vi "Write Error Log.vi"(5 "system directory type":T1=1 items=["User Home"=0, "User Desktop"=1, "User Documents"=2, "User Application Data"=3, "User Preferences"=4, "User Temporary"=5, "Public Documents"=6, "Public Application Data"=7, "Public Preferences"=8, "Public Cache"=13, "System Core Libraries"=9, "System Installed Libraries"=10, "Application Files"=11, "Boot Volume Root"=12], 6 "Thread":string, 7 "error IO":errorcluster, 9 "Additional info":string) -> (0 "error out":errorcluster)   [LabVIEW 2017]
uses:
  <vilib>/Utility/sysdir.llb/System Directory Type.ctl
  <vilib>/Utility/error.llb/DialogType.ctl
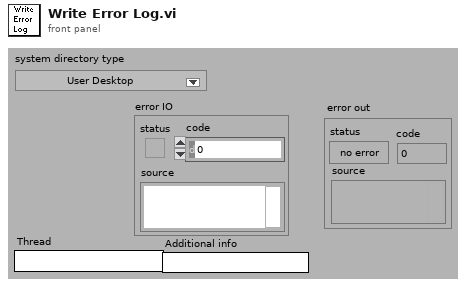
[diagram p1: front panel]
types:
  T1 = typedef "System Directory Type.ctl" = i32
  T2 = typedef "DialogType.ctl" = u16
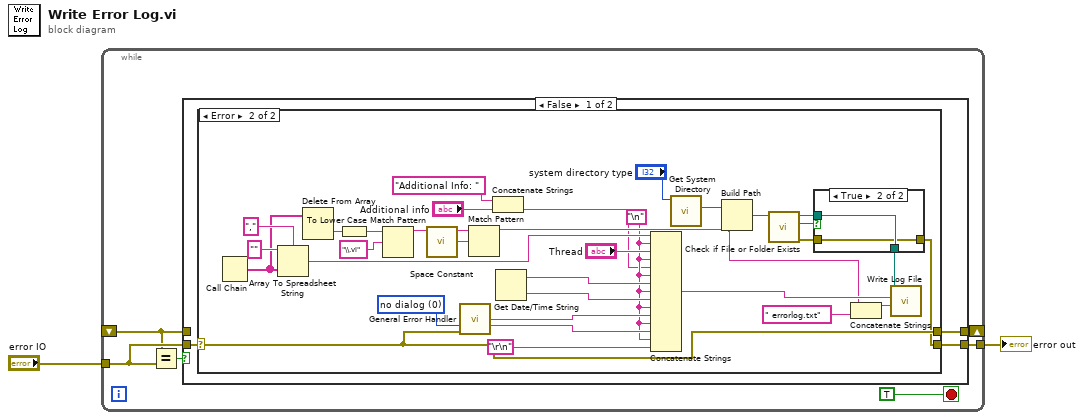
[diagram p0: block diagram]
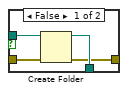
[diagram p3: hidden frame]
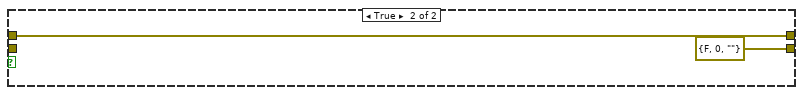
[diagram p4: hidden frame]
diagram:
  n1 = while {
    shift-right: [w8] -> _
    shift-left: _ -> [w4]
    tunnel: "error IO" -> [w5]
    tunnel: [w3] -> w1
    stop <- TRUE stop-if-true
    n2 = Equal?(x=w4, y=w5) -> (x = y?=w6:bool)
    n3 = case shown="False" w6 {
      tunnel: [w10 w53] -> w8
      tunnel: w5 -> [w11 _]
      tunnel: w4 -> [_ w53]
      tunnel: [w9 errorcluster {"status"=FALSE, "code"=0, "source"=""} ("error IO")] -> w3
      frame False {
        n4 = case shown="Error" w11 {
          selector: w11 -> [w12 w35]
          tunnel: [w12 w35] -> w10
          tunnel: [w12 w29] -> w9
          frame No Error {
          }
          frame Error {
            w40 = T2 0 items=["no dialog", "OK message", "continue or stop message", "OK message + warnings", "continue/stop + warnings"] ("type of dialog (OK msg:1)")
            w14 = "\n"
            n5 = Call Chain() -> (call chain=w26:string[])
            n6 = Array To Spreadsheet String(delimiter (Tab)=",", array=w26, 3:"" ("format string")) -> (spreadsheet string=w22:string)
            n7 = Delete From Array(array=w26) -> (deleted portion=w25:string)  [unwired: 2 in, 1 out]
            n8 = To Lower Case(string=w25) -> (all lower case string=w23:string)
            n9 = Match Pattern(string=w23, regular expression="\\.vi") -> (before substring=w20:string)  [unwired: 1 in, 3 out]
            n10 = call <vilib>:"Space Constant.vi"() -> ("String"=w19:string)
            n11 = call <vilib>:"General Error Handler.vi"("type of dialog (OK msg:1)"=w40, "error in (no error)"=w35) -> ("source out"=w43:string, "message"=w44:string)  [unwired: 1 in, 11 out]
            n12 = Match Pattern(string=w20, regular expression=w19) -> (before substring=w18:string)  [unwired: 1 in, 3 out]
            n13 = Concatenate Strings("Additional Info: " ("string"), "Additional info") -> (w13:string)
            n14 = Get Date/Time String() -> (date string=w41:string, time string=w42:string)  [unwired: 3 out]
            n15 = Concatenate Strings(w22, w14, "Thread", w14, w13, w14, w41, w14, w42, w14, w43, w14, w44, w14, "\r\n") -> (w45:string)
            n16 = call <vilib>:"Get System Directory.vi"("system directory type"="system directory type") -> ("system directory"=w37:path)  [unwired: 10 in]
            n17 = Build Path(base path=w37, name or relative path=w18) -> (appended path=w34:path)
            n18 = call <vilib>:"Check if File or Folder Exists.vi"("path"=w34) -> ("error out"=w30:errorcluster, "file or folder exists?"=w33:bool, "dup path"=w32:path)  [unwired: 8 in]
            n19 = case shown="True" w33 {
              tunnel: w32 -> [w49 w51]
              tunnel: [w48 w51] -> w31
              tunnel: w30 -> [w47 w50]
              tunnel: [w46 w50] -> w29
              frame False {
                n20 = Create Folder(path (use dialog)=w49, error in=w47) -> (created path=w48:path, error out=w46:errorcluster)  [unwired: 1 in, 1 out]
              }
              frame True {
              }
            }
            n21 = Concatenate Strings(w18, " errorlog.txt" ("name or relative path")) -> (w36:string)
            n22 = call "Write Log File .vi"("filename"=w36, "String to Append"=w45, "base path"=w31) -> ()  [unwired: 8 in, 1 out]
          }
        }
      }
      frame True {
      }
    }
  }
  "error out" <- w1
